vi "PH_ForceSensor.destructor.vi"(0 "i ref in":refnum<vi>, 5 "error in(no error)":errorcluster) -> (19 "error out":errorcluster)   [LabVIEW 2014, in "PH_ForceSensor.lvlib"]
doc: "This is the destructor of a class.\n\nLicense Agreement for this software:\n\nCopyright (C)\nGesellschaft für Schwerionenforschung, GSI\nPlanckstr. 1\n64291 Darmstadt\nGermany\n\nContact: D.Beck@gsi.de \n\nThis program is free software; you can redistribute it and/or modify it under the terms of the \nGNU General Public License as published by the Free Software Foundation; either version 2 of \nthe license, or (at your option) any later version.\n\nThis program is distributed in the hope that it will be useful, but WITHOUT ANY WARRANTY; \nwithout even the implied warranty of MERCHANTABILITY or FITNESS FOR A PARTICULAR PURPOSE. See the GNU General License for more details (http://www.gnu.org).\n\nGesellschaft für Schwerionenforschung, GSI\nPlanckstr. 1, 64291 Darmstadt, Germany\nFor all questions and ideas contact: M.Richter@gsi.de, H.Brand@gsi.de or D.Beck@gsi.de.\nLast update: 16-JUN-2004"
uses:
  PH_ForceSensor.lvlib
  PH_Basics/PH_PSDBWriter/PH_PSDBWriter.lvlib
  PHELIX/PH_BeamlineInformation/PH_BeamlineInformation.lvlib
  PH_Basics/PH_StatusHandler/PH_StatusHandler.lvlib
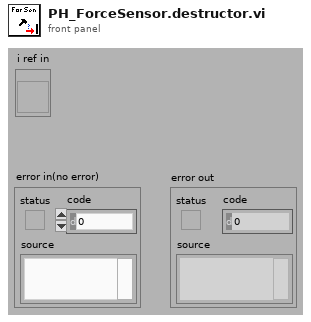
[diagram p1: front panel]
types:
  T1 = typedef "PH_ForceSensor.lvlib/PH_ForceSensor.i attribute.ctl" = cluster{"GUI Refs":T2, "Rawvalues":T3, "Offsets [µV]":T3, "Scalings [mV/V]":T3, "Forces [N]":T3, "Supply Voltage [V]":dbl, "Full Force [N]":dbl, "Ranges [N]":cluster{"Low Energy":cluster{"Upper Limit":dbl, "Lower Limit":dbl}, "High Energy":cluster{"Upper Limit":dbl, "Lower Limit":dbl}}}
  T2 = typedef "PH_ForceSensor.lvlib/PH_ForceSensor.GUI Refs.ctl" = cluster{"Delete":refnum<vi>, "Rawvalues":refnum<vi>, "Offsets [µV]":refnum<vi>, "Sensor Values [µV]":refnum<vi>, "Scalings [mV/V]":refnum<vi>, "Supply Voltage [V]":refnum<vi>, "Full Force [N]":refnum<vi>, "Forces [N]":refnum<vi>, "Graph Differential Forces":refnum<vi>, "Graph Absolute Forces":refnum<vi>, "Ranges [N]":refnum<vi>}
  T3 = typedef "PH_ForceSensor.lvlib/PH_ForceSensor.Dataset.ctl" = cluster{"top front":dbl, "top back":dbl, "bottom front":dbl, "bottom back":dbl}
  T4 = enum16{"SetAttribute", "GetAttribute", "CreateAttribute", "DestroyAttribute", "DestroyAllAtributes"}
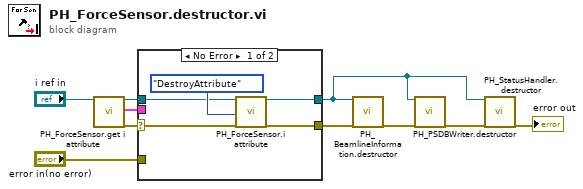
[diagram p0: block diagram]
diagram:
  n1 = call "PH_ForceSensor.get i attribute.vi"("i ref in"="i ref in") -> ("i ref out"=w9:refnum<vi>, "i attribute"=w8:T1, "error out"=w7:errorcluster)  [unwired: 16 in]
  n2 = case shown="No Error" w7 {
    selector: w7 -> [w11 _]
    tunnel: [w14 w16] -> w5
    tunnel: w9 -> [w13 w17]
    tunnel: w8 -> [_ _]
    tunnel: [w12 w17] -> w1
    tunnel: "error in(no error)" -> [_ w16]
    frame No Error {
      n3 = call "PH_ForceSensor.i attribute.vi"("VI Refnum"=w13, "Action"=T4."DestroyAttribute", "error in (no error)"=w11) -> ("VI Refnum out"=w12:refnum<vi>, "error out"=w14:errorcluster)  [unwired: 14 in, 1 out]
    }
    frame Error {
    }
  }
  n4 = call "PH_BeamlineInformation.destructor.vi"("i ref in"=w1, "error in(no error)"=w5) -> ("error out"=w3:errorcluster)  [unwired: 17 in]
  n5 = call "PH_PSDBWriter.destructor.vi"("i ref in"=w1, "error in(no error)"=w3) -> ("error out"=w4:errorcluster)  [unwired: 17 in]
  n6 = call "PH_StatusHandler.destructor.vi"("i ref in"=w1, "error in(no error)"=w4) -> ("error out"=→"error out":errorcluster)  [unwired: 17 in]
